vi "Color Selector.vi"(11 "Numeric Control":dbl) -> (3 "Color Box":u32(colorbox))   [LabVIEW 2015]
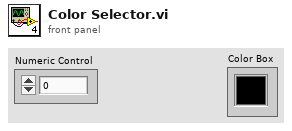
[diagram p1: front panel]
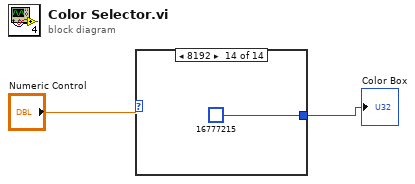
[diagram p0: block diagram]
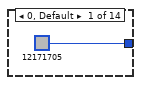
[diagram p2: hidden frame]
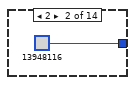
[diagram p3: hidden frame]
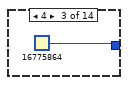
[diagram p4: hidden frame]
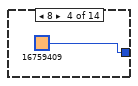
[diagram p5: hidden frame]
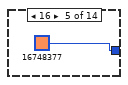
[diagram p6: hidden frame]
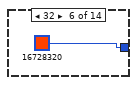
[diagram p7: hidden frame]
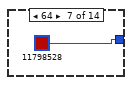
[diagram p8: hidden frame]
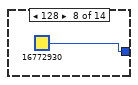
[diagram p9: hidden frame]
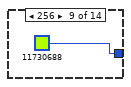
[diagram p10: hidden frame]
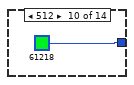
[diagram p11: hidden frame]
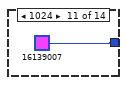
[diagram p12: hidden frame]
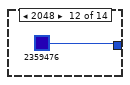
[diagram p13: hidden frame]
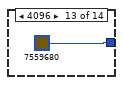
[diagram p14: hidden frame]
diagram:
  n1 = case shown="8192" "Numeric Control" {
    tunnel: [u32 12171705 u32 13948116 u32 16775864 u32 16759409 u32 16748377 u32 16728320 u32 11798528 u32 16772930 u32 11730688 u32 61218 u32 16139007 u32 2359476 u32 7559680 u32 16777215] -> w1
    frame 0, Default {
    }
    frame 2 {
    }
    frame 4 {
    }
    frame 8 {
    }
    frame 16 {
    }
    frame 32 {
    }
    frame 64 {
    }
    frame 128 {
    }
    frame 256 {
    }
    frame 512 {
    }
    frame 1024 {
    }
    frame 2048 {
    }
    frame 4096 {
    }
    frame 8192 {
    }
  }
  "Color Box" <- w1
